vi "sc_store.vi"(1 "Previous":bool, 2 "Data":dbl, 3 "Ack":bool) -> (0 "Boolean":bool)   [LabVIEW 2017]
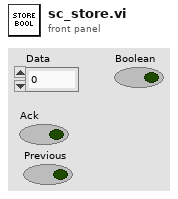
[diagram p1: front panel]
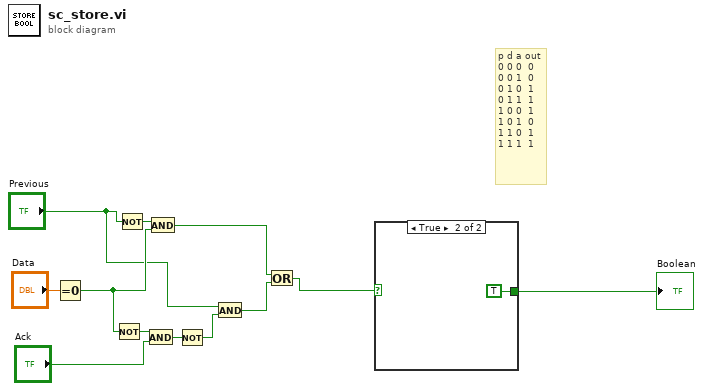
[diagram p0: block diagram]
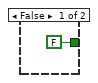
[diagram p2: hidden frame]
diagram:
  # "p d a out\n0 0 0  0\n0 0 1  0\n0 1 0  1\n0 1 1  1\n1 0 0  1\n1 0 1  0\n1 1 0  1\n1 1 1  1"
  n1 = Equal To 0?(x="Data") -> (x = 0?=w7:bool)
  n2 = Not(x=w7) -> (.not. x?=w8:bool)
  n3 = Not(x="Previous") -> (.not. x?=w10:bool)
  n4 = And(x=w8, y="Ack") -> (x .and. y?=w9:bool)
  n5 = And(x=w10, y=w7) -> (x .and. y?=w2:bool)
  n6 = Not(x=w9) -> (.not. x?=w5:bool)
  n7 = And(x="Previous", y=w5) -> (x .and. y?=w3:bool)
  n8 = Or(x=w2, y=w3) -> (x .or. y?=w1:bool)
  n9 = case shown="True" w1 {
    tunnel: [FALSE TRUE] -> w11
    frame False {
    }
    frame True {
    }
  }
  "Boolean" <- w11
